vi "SVT Fractional Octave Filtering (1 Ch).vi"(6 "reset filter (F)":bool, 7 "coerce to nearest standard midband frequency?":bool, 8 "error in (no error)":errorcluster, 9 "midband frequency":dbl, 10 "bandwidth":T1(ring), 11 "scaled signal [EU]":waveform(dbl)) -> (0 "error out":errorcluster, 2 "actual midband frequency [Hz]":dbl, 3 "filtered signal [EU]":waveform(dbl), 4 "settled?":bool)   [LabVIEW 2017, in "SoundVib_Octave_2014 standard.lvlib"]
doc: "Performs fractional octave filtering on <B>scaled signal [EU]</B> in accordance with either the ANSI S1.11-2014 standard or the IEC 61260-1:2014 standard.\n\n \n\nYou can use this polymorphic VI to perform fractional octave filtering on a single channel or on N channels. The data type you wire to the <B>scaled signal [EU]</B> input determines the polymorphic instance to use."
uses:
  <vilib>/addons/Sound and Vibration/svt_Octave/SoundVib_Octave_2014 standard.lvlib
  <vilib>/addons/_NISVFA/_Shared subVIs/Controls/svc_Octave Standard.ctl
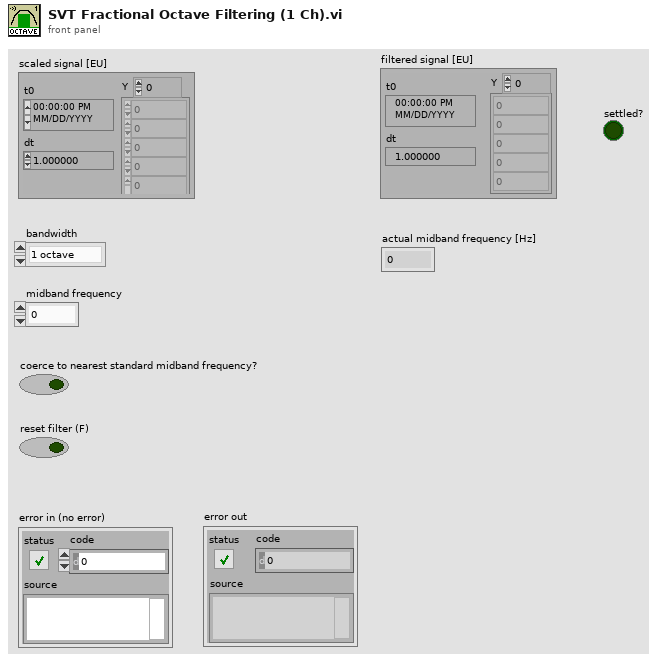
[diagram p1: front panel]
types:
  T1 = enum16{"1 octave", "1/3 octave", "1/6 octave", "1/12 octave", "1/24 octave"}
  T2 = typedef "svc_Octave Standard.ctl" = enum16{"ANSI S1.11", "IEC 61260"}
  T3 = cluster{"standard":T2, "bandwidth":enum16{"1 octave", "1/3 octave", "1/6 octave", "1/12 octave", "1/24 octave"}}
  T4 = cluster{"midband frequency":dbl, "coerce to nearest standard midband frequency?":bool}
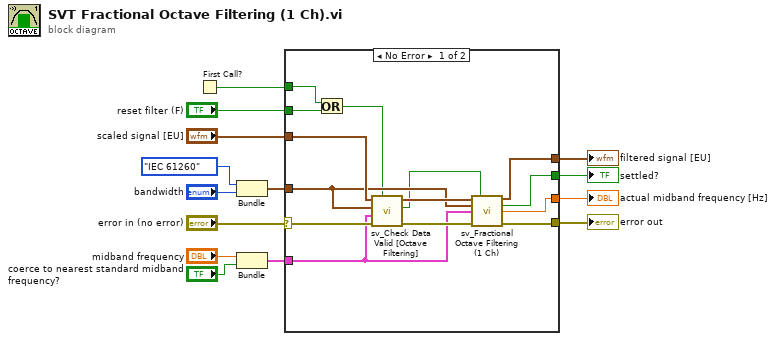
[diagram p0: block diagram]
diagram:
  n1 = First Call?() -> (First Call?: T/F=w8:bool)
  n2 = Bundle("standard"=svc_Octave_Standard."IEC 61260", "bandwidth"="bandwidth") -> (w1:T3)  [unwired: 1 in]
  n3 = Bundle("midband frequency"="midband frequency", "coerce to nearest standard midband frequency?"="coerce to nearest standard midband frequency?") -> (w4:T4)  [unwired: 1 in]
  n4 = case shown="No Error" "error in (no error)" {
    selector: "error in (no error)" -> [w26 w29]
    tunnel: [w24 w29] -> w13
    tunnel: "scaled signal [EU]" -> [w23 _]
    tunnel: "reset filter (F)" -> [w18 _]
    tunnel: [w28 _] -> w9
    tunnel: [w27 _] -> w10
    tunnel: w1 -> [w21 _]
    tunnel: w4 -> [w20 _]
    tunnel: w8 -> [w16 _]
    tunnel: [w15 _] -> w7
    frame No Error {
      n5 = Or(x=w16, y=w18) -> (x .or. y?=w17:bool)
      n6 = call <vilib>:"sv_Check Data Valid [Octave Filtering].vi"("reset filter (F)"=w17, "error in (no error)"=w26, "midband frequency setting"=w20, "1/n octave settings"=w21, "scaled signal [EU]"=w23) -> ("error out"=w25:errorcluster, "reset filter"=w19:bool, "dup scaled signal [EU]"=w22:waveform(dbl))  [unwired: 4 in]
      n7 = call <vilib>:"sv_Fractional Octave Filtering (1 Ch).vi"("scaled signal [EU]"=w22, "reset filter (F)"=w19, "1/n octave settings"=w21, "midband frequency setting"=w20, "error in (no error)"=w25) -> ("filtered signal [EU]"=w27:waveform(dbl), "settled?"=w28:bool, "actual midband frequency [Hz]"=w15:dbl, "error out"=w24:errorcluster)  [unwired: 7 in]
    }
    frame Error {
    }
  }
  "error out" <- w13
  "filtered signal [EU]" <- w10
  "settled?" <- w9
  "actual midband frequency [Hz]" <- w7
